vi "Launch Model.vi"(8 "error in (no error)":errorcluster, 11 "IViewModel In":refnum<class "IViewModel.lvclass">) -> (0 "error out":errorcluster, 3 "IViewModel Out":refnum<class "IViewModel.lvclass">)   [LabVIEW 2015, in "IViewModel.lvlib" / "IViewModel.lvclass"]
doc: "<License>\nCopyright © 2017 Composed Systems, LLC | All rights reserved\nwww.composed.io\n\nAuthor: Ethan Stern <ethan.stern@composed.io>\n\nThis software is provided \"AS IS\" WITHOUT WARRANTIES, either express or implied, AND IS FOR EDUCATIONAL PURPOSES ONLY.\n</License>"
uses:
  IViewModel.lvclass
  IViewModel.lvclass/IViewModel.ctl
  IMediator/IMediator Messages/Publish Msg/Publish Msg.lvclass
  IMediator/IMediator Messages/Subscribe Msg/Subscribe Msg.lvclass
  AbstractMessages/PreAddressedMsg/PreAddressedMsg.lvclass/PreAddressedMsg.ctl
  IModel/IModel/IModel.lvclass/IModel.ctl
  <vilib>/ActorFramework/Actor/Actor.lvclass
  IModel/IModel/IModel.lvclass
  AbstractMessages/PreAddressedMsg/PreAddressedMsg.lvclass
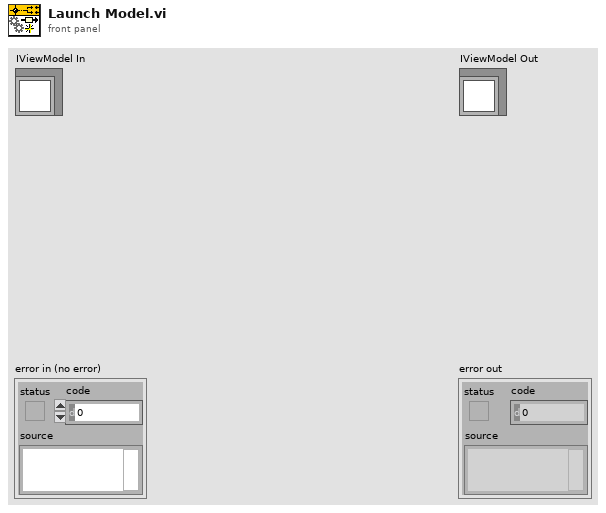
[diagram p1: front panel]
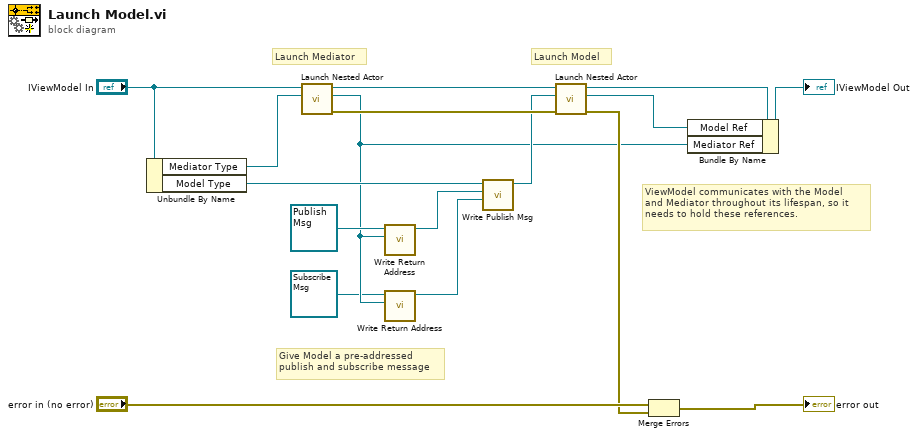
[diagram p0: block diagram]
diagram:
  # "Launch Model"
  # "Launch Mediator"
  # "Give Model a pre-addressed\npublish and subscribe message"
  # "ViewModel communicates with the Model\nand Mediator throughout its lifespan, so it\nneeds to hold these references."
  n1 = Unbundle By Name("IViewModel In") -> ("Mediator Type"=w14:refnum<class "IMediator.lvclass">, "Model Type"=w13:refnum<class "IModel.lvclass">)
  n2 = call <vilib>:"Launch Nested Actor.vi"("Nested Actor"=w14, "Caller Actor in"="IViewModel In") -> ("error out"=w9:errorcluster, "Nested Actor's Enqueuer"=w3:refnum<class "Message Enqueuer.lvclass">, "Caller Actor out"=w15:refnum<class "IViewModel.lvclass">)  [unwired: 7 in]
  n3 = call "Write Return Address.vi"("Return Address"=w3, "PreAddressedMsg in"=refnum<class "Publish Msg.lvclass"> refnum ("IMediator.lvlib:Publish Msg.lvclass")) -> ("PreAddressedMsg out"=w5:refnum<class "Publish Msg.lvclass">)  [unwired: 9 in]
  n4 = call "Write Return Address.vi"("Return Address"=w3, "PreAddressedMsg in"=refnum<class "Subscribe Msg.lvclass"> refnum ("IMediator.lvlib:Subscribe Msg.lvclass")) -> ("PreAddressedMsg out"=w1:refnum<class "Subscribe Msg.lvclass">)  [unwired: 9 in]
  n5 = call "Write Publish Msg.vi"("Pre-Addressed Subscribe Msg"=w1, "Pre-Addressed Publish Msg"=w5, "IModel in"=w13) -> ("IModel out"=w6:refnum<class "IModel.lvclass">)  [unwired: 8 in]
  n6 = call <vilib>:"Launch Nested Actor.vi"("error in (no error)"=w9, "Nested Actor"=w6, "Caller Actor in"=w15) -> ("error out"=w7:errorcluster, "Nested Actor's Enqueuer"=w10:refnum<class "Message Enqueuer.lvclass">, "Caller Actor out"=w12:refnum<class "IViewModel.lvclass">)  [unwired: 6 in]
  n7 = Merge Errors("error in (no error)", w7) -> (→"error out":errorcluster)
  n8 = Bundle By Name(cluster=w12, "Model Ref"=w10, "Mediator Ref"=w3) -> (→"IViewModel Out":refnum<class "IViewModel.lvclass">)
